vi "EnableDisable RTM.vi"(8 "error in (no error)":errorcluster, 11 "Node Ptr":u64 format="%.0x") -> (0 "error out":errorcluster)   [LabVIEW 2020, in "AIM MIL-STD-1553 System Explorer.lvlib" / "Implementation.lvlib"]
uses:
  Implementation.lvlib
  Scripting/AIM MIL-STD-1553 Scripting.lvlib
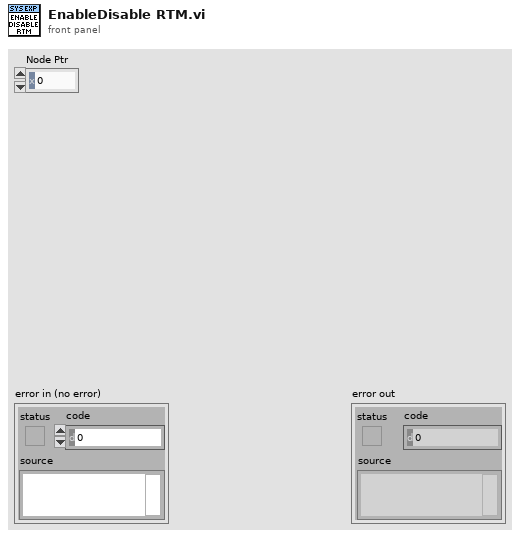
[diagram p1: front panel]
types:
  T1 = typedef "Custom Device API.lvlib/Custom Device Item Ref.ctl" = u64
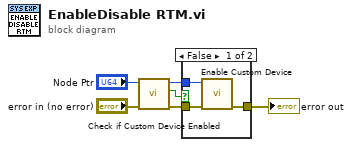
[diagram p0: block diagram]
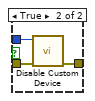
[diagram p2: hidden frame]
diagram:
  n1 = call "Check if Custom Device Enabled.vi"("error in"="error in (no error)", "custom device ref in"="Node Ptr") -> ("error out"=w4:errorcluster, "Custom Device is Enabled"=w1:bool, "custom device ref out"=w5:T1)  [unwired: 7 in]
  n2 = case shown="False" w1 {
    tunnel: w5 -> [w9 w10]
    tunnel: w4 -> [w8 w12]
    tunnel: [w7 w11] -> w2
    frame False {
      n3 = call "Enable Custom Device.vi"("error in"=w8, "custom device ref in"=w9) -> ("error out"=w7:errorcluster)  [unwired: 8 in, 1 out]
    }
    frame True {
      n4 = call "Disable Custom Device.vi"("error in"=w12, "custom device ref in"=w10) -> ("error out"=w11:errorcluster)  [unwired: 8 in, 1 out]
    }
  }
  "error out" <- w2
